vi "Load and Open All Items.vi"(8 "error in (no error)":errorcluster, 11 "Application Data in":T1 {"current buffer data"."channels"."configuration"."string offset" format="%d bytes"; "current buffer data"."avg bandwidth" format="%.0g bytes"}) -> (0 "error out":errorcluster, 3 "Application Data out":T1 {"current buffer data"."channels"."configuration"."string offset" format="%d bytes"; "current buffer data"."avg bandwidth" format="%.0g bytes"})   [LabVIEW 2017, in "Data Viewer.lvlib"]
uses:
  Core/VIs/Data Viewer/Source/Data Viewer.lvlib
  Application Data.ctl
  <vilib>/NI/Memory Manager/Classes/Pointer/Pointer.lvclass
  VeriStand/Data Sharing Custom Device/Source/DSF Core.lvlibp/Classes/Configuration/Core/Framework/Framework Configuration.lvclass
  Buffer Reader/Queue Data.ctl
  Buffer Reader/Buffer Data.ctl
  VeriStand/Data Sharing Custom Device/Source/DSF Core.lvlibp/Classes/Configuration/Core/Transfer/Channel Configuration.ctl
  VeriStand/Data Sharing Custom Device/Source/DSF Core.lvlibp/Typedefs/Core Channel Configuration.ctl
  VeriStand/Data Sharing Custom Device/Source/DSF Core.lvlibp/Typedefs/DSF Data Type.ctl
  VeriStand/Data Sharing Custom Device/Source/DSF Core.lvlibp/Typedefs/DSF Settings Info.ctl
  VeriStand/Data Sharing Custom Device/Source/DSF Core.lvlibp/Typedefs/DSF Byte Order.ctl
  VeriStand/Data Sharing Custom Device/Source/DSF Core.lvlibp/Classes/Thread/Data Server/DSF Buffer Subset Descriptor.ctl
  VeriStand/Data Sharing Custom Device/Source/DSF Core.lvlibp/Typedefs/DSF Buffer Type.ctl
  Values Channels.ctl
  VeriStand/Data Sharing Custom Device/Source/DSF Core.lvlibp
  VeriStand/Data Sharing Custom Device/Source/DSF Core.lvlibp/Classes/Configuration/Core/Channel/Channel Configuration.lvclass
  VeriStand/Data Sharing Custom Device/Source/DSF Core.lvlibp/Classes/Configuration/Core/Transfer/Transfer Configuration.lvclass
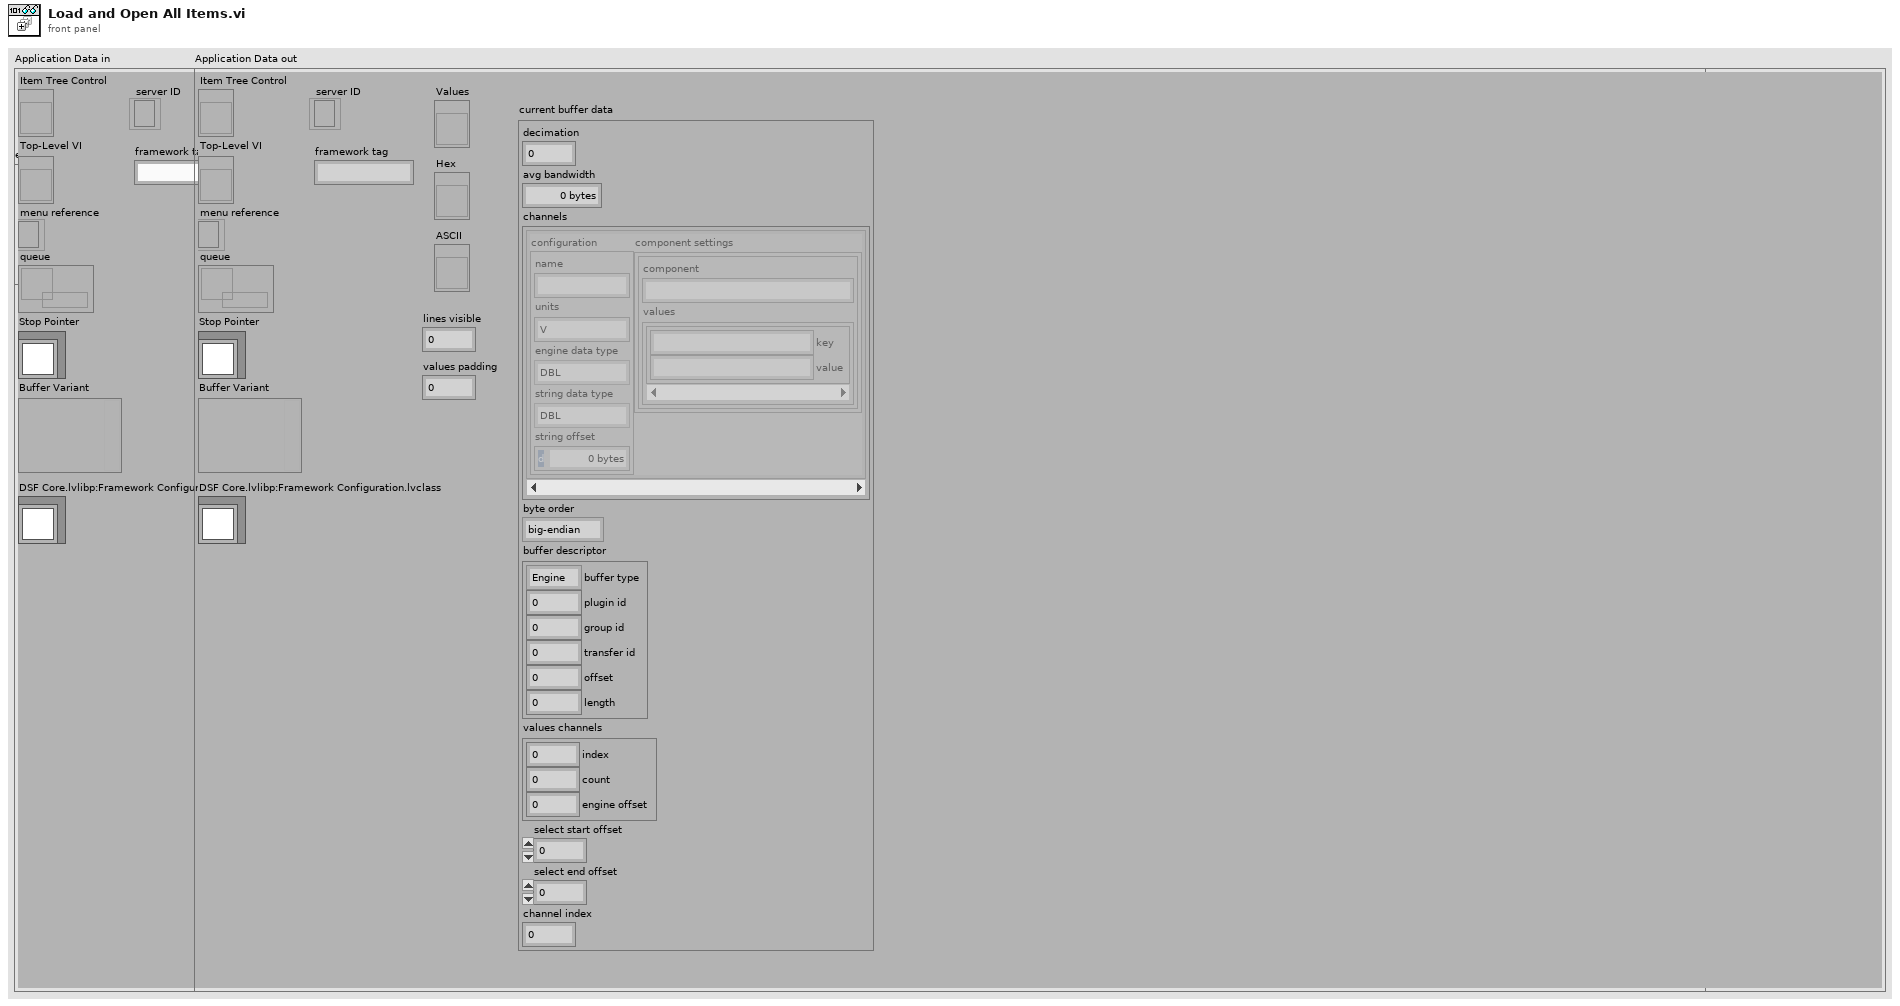
[diagram p1: front panel]
types:
  T1 = typedef "Data Viewer.lvlib/Application Data.ctl" = cluster{"Item Tree Control":refnum<vi>, "Top-Level VI":refnum<vi>, "menu reference":refnum<k9>, "queue":refnum<queue>, "Stop Pointer":refnum<class "Pointer.lvclass">, "Buffer Variant":variant, "server ID":refnum<k5>, "framework tag":string, "Values":refnum<vi>, "Hex":refnum<vi>, "ASCII":refnum<vi>, "lines visible":i32, "values padding":i32, "current buffer data":T2, "DSF Core.lvlibp:Framework Configuration.lvclass":refnum<class "Framework Configuration.lvclass">}
  T2 = typedef "Data Viewer.lvlib/Buffer Data.ctl" = cluster{"decimation":u64, "avg bandwidth":dbl, "channels":T3[], "byte order":T7, "buffer descriptor":T8, "values channels":T10, "select start offset":u64, "select end offset":u64, "channel index":i32}
  T3 = typedef "DSF Core.lvlibp/Transfer Configuration.lvclass/Channel Configuration.ctl" = cluster{"configuration":T4, "component settings":T6[]}
  T4 = typedef "DSF Core.lvlibp/Channel Configuration.lvclass/Core Channel Configuration.ctl" = cluster{"name":string, "units":string, "engine data type":T5, "string data type":T5, "string offset":u64}
  T5 = typedef "DSF Core.lvlibp/DSF Data Type.ctl" = enum8{"Bool", "SGL", "DBL", "I8", "I16", "I32", "I64", "U8", "U16", "U32", "U64"}
  T6 = typedef "DSF Core.lvlibp/DSF Settings Info.ctl" = cluster{"component":string, "values":cluster{"key":string, "value":string}[]}
  T7 = typedef "DSF Core.lvlibp/DSF Byte Order.ctl" = enum8{"big-endian", "little-endian"}
  T8 = typedef "DSF Core.lvlibp/DSF Buffer Subset Descriptor.ctl" = cluster{"buffer type":T9, "plugin id":i32, "group id":i32, "transfer id":i32, "offset":u64, "length":i64}
  T9 = typedef "DSF Core.lvlibp/DSF Buffer Type.ctl" = enum16{"Engine", "String"}
  T10 = typedef "Data Viewer.lvlib/Values Channels.ctl" = cluster{"index":i32, "count":i32, "engine offset":u64}
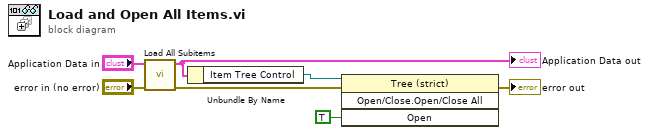
[diagram p0: block diagram]
diagram:
  n1 = call "Load All Subitems.vi"("error in (no error)"="error in (no error)", "Application Data in"="Application Data in") -> ("error out"=w1:errorcluster, "Application Data out"=w4:T1)  [unwired: 8 in]
  "Application Data out" <- w4
  n2 = Unbundle By Name(w4) -> ("Item Tree Control"=w6:refnum<vi>)
  n3 = invoke class="Tree (strict)" method="Open/Close.Open/Close All"(reference=w6, error in=w1, "Open"=TRUE ("Open?")) -> (error out=→"error out":errorcluster)  [unwired: 1 in, 3 out]
